vi "关闭SIEMENS.vi"(8 "error in (no error)":errorcluster caption="错误输入（无错误）", 11 "gInitialSIEMENSS7 In":refnum<k24>) -> (0 "error out":errorcluster caption="错误输出")   [LabVIEW 2017]
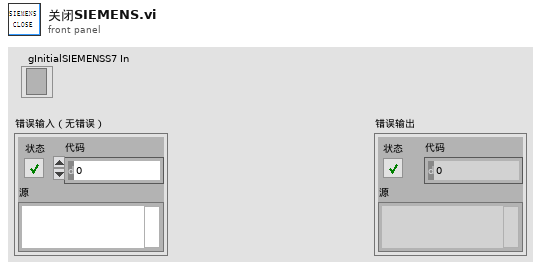
[diagram p1: front panel]
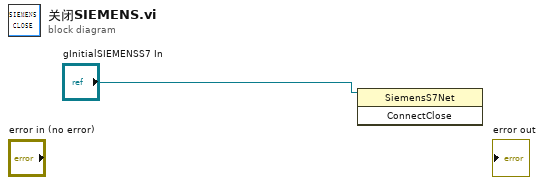
[diagram p0: block diagram]
diagram:
  n1 = invoke class="SiemensS7Net" method="ConnectClose"(reference="gInitialSIEMENSS7 In") -> ()  [unwired: 2 in, 3 out]
